vi "TCPServer.vi"() -> ()   [LabVIEW 2015]
uses:
  SystemUtil/Command.ctl
  Log/LogItem.ctl
  TCPServer_Global.vi
panel:
  in  "CommandQ":string
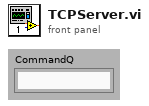
[diagram p1: front panel]
types:
  T1 = typedef "Command.ctl" = cluster{"Command":string, "Parameter":string}
  T2 = typedef "LogItem.ctl" = cluster{"error in (no error)":errorcluster, "Source":string, "Comment ":string}
  T3 = enum16{"Launch", "Log", "Open", "Close", "Shutdown"}
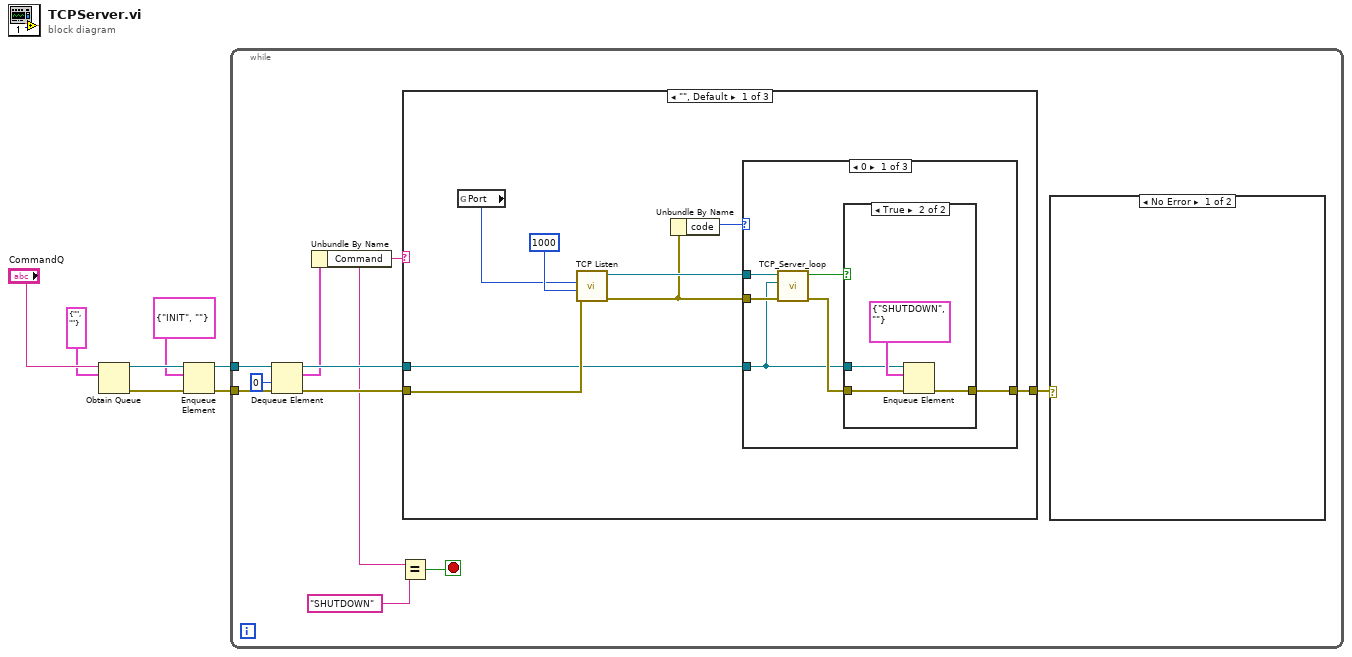
[diagram p0: block diagram]
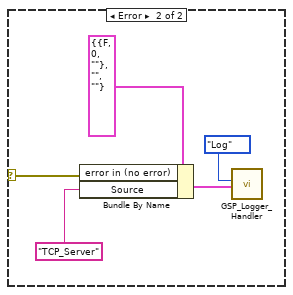
[diagram p2: hidden frame]
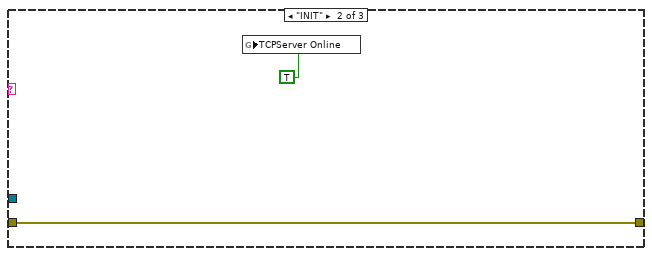
[diagram p6: hidden frame]
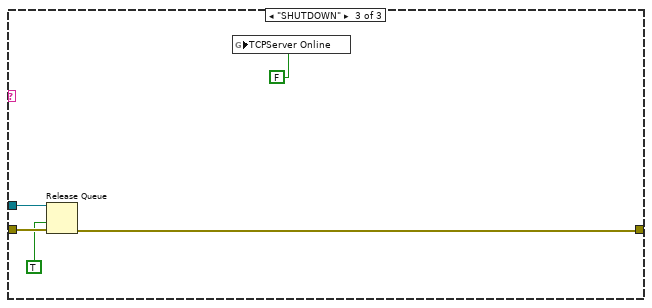
[diagram p7: hidden frame]
diagram:
  n1 = Obtain Queue(name (unnamed)="CommandQ", element data type=T1 {"Command"="", "Parameter"=""} ("Command")) -> (queue out=w3:refnum<queue>, error out=w2:errorcluster)  [unwired: 3 in, 1 out]
  n2 = Enqueue Element(queue=w3, element=T1 {"Command"="INIT", "Parameter"=""}, error in (no error)=w2) -> (queue out=w5:refnum<queue>, error out=w4:errorcluster)  [unwired: 1 in, 1 out]
  n3 = while {
    tunnel: w5 -> [w17]
    tunnel: w4 -> [w16]
    stop <- w9 stop-if-true
    n4 = Dequeue Element(queue=w17, timeout in ms (-1)=0, error in (no error)=w16) -> (queue out=w15:refnum<queue>, element=w13:T1, error out=w14:errorcluster)  [unwired: 1 out]
    n5 = Unbundle By Name(w13) -> ("Command"=w11:string)
    n6 = Equal?(x=w11, y="SHUTDOWN") -> (x = y?=w9:bool)
    n7 = case shown="\"\", Default" w11 {
      tunnel: w15 -> [w26 _ w48]
      tunnel: w14 -> [w28 w42 w47]
      tunnel: [w25 w42 w45] -> w8
      frame "", Default {
        n8 = global read "TCPServer_Global.vi" "Port"() -> (w27:u16)
        n9 = call <vilib>:"TCP Listen.vi"("error in (no error)"=w28, "timeout ms (wait forever: -1)"=1000, "port"=w27) -> ("error out"=w23:errorcluster, "connection ID"=w24:refnum<k5>)  [unwired: 4 in, 3 out]
        n10 = Unbundle By Name(w23) -> ("code"=w30:i32)
        n11 = case shown="0" w30 {
          tunnel: w24 -> [w36 _ _]
          tunnel: w23 -> [w35 _ _]
          tunnel: w26 -> [w31 _ _]
          tunnel: [w32 _ _] -> w25
          frame 0 {
            n12 = call "TCP_Server_loop.vi"("error in (no error)"=w35, "queue in"=w31, "TCP Connection ID"=w36) -> ("error out"=w33:errorcluster, "Shutdown?"=w34:bool)  [unwired: 3 in]
            n13 = case shown="True" w34 {
              tunnel: w33 -> [w37 w41]
              tunnel: [w37 w40] -> w32
              tunnel: w31 -> [_ w38]
              frame False {
              }
              frame True {
                n14 = Enqueue Element(queue=w38, element=T1 {"Command"="SHUTDOWN", "Parameter"=""}, error in (no error)=w41) -> (error out=w40:errorcluster)  [unwired: 1 in, 2 out]
              }
            }
          }
          frame 1, Default {
          }
          frame 56 {
          }
        }
      }
      frame "INIT" {
        n15 = global write "TCPServer_Global.vi" "TCPServer Online"(TRUE) -> ()
      }
      frame "SHUTDOWN" {
        n16 = Release Queue(queue=w48, force destroy? (F)=TRUE, error in (no error)=w47) -> (error out=w45:errorcluster)  [unwired: 2 out]
        n17 = global write "TCPServer_Global.vi" "TCPServer Online"(FALSE) -> ()
      }
    }
    n18 = case shown="No Error" w8 {
      selector: w8 -> [_ w18]
      frame No Error {
      }
      frame Error {
        n19 = Bundle By Name(cluster=T2 {"error in (no error)"={"status"=FALSE, "code"=0, "source"=""}, "Source"="", "Comment "=""} ("Log"), "error in (no error)"=w18, "Source"="TCP_Server") -> (w21:T2)
        n20 = call "GSP_Logger_Handler.vi"("Log"=w21, "Actions"=T3."Log") -> ()  [unwired: 5 in, 1 out]
      }
    }
  }
